vi "StateMachineOperation.vi"() -> ()   [LabVIEW 2020]
panel:
  out "First Ball Color AJ":string
  out "Shooter Eject":bool
  out "Second Ball Color":string
  out "First Ball Color":string
  out "Opposite Color":string
  out "Ball Color":string
  out "Climber - Reset":bool
  out "Climber - Pull":bool
  out "Enable Shooter":bool
  # "Shooter"
  # "Conveyor"
  # "Climber"
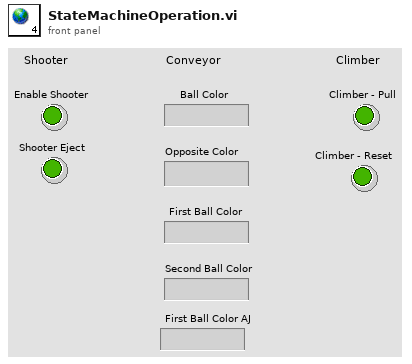
[diagram p1: front panel]
diagram:
